vi "Convolutional_perso.vi"() -> ()   [LabVIEW 2018]
uses:
  <vilib>/Analysis/1siggen.llb/Ramp Pattern by Samples.vi
  <vilib>/addons/Modulation/Digital/General/MT Generate Bits (Galois, PN Order).vi
  <vilib>/addons/Modulation/Digital/Channel Coding/MT Convolutional Encoder (Rate).vi
  <vilib>/Analysis/baseanly.llb/Mean (DBL).vi
  <vilib>/addons/Modulation/Analog/support/mod_Set Error Source.vi
  <vilib>/addons/Modulation/Digital/Support/Common/Validators/mod_Generate Bits Validate.vi
  <vilib>/addons/Modulation/Digital/Support/Common/Validators/mod_Validate Bit Stream.vi
  <vilib>/addons/Modulation/Digital/Channel Coding/Convolutional codes/mod_Convolutional encoder.vi
  <vilib>/addons/Modulation/Digital/Support/Common/Validators/mod_AWGN Validate.vi
  <vilib>/addons/Modulation/Digital/Impairments/subVIs/mod_createSeeds.vi
  <vilib>/addons/Modulation/Digital/Channel Coding/Convolutional codes/subVIs/mod_Generate encoder tap connections.vi
  <vilib>/addons/Modulation/Digital/Channel Coding/Convolutional codes/subVIs/mod_Perform convolutional encoding.vi
  <vilib>/addons/Modulation/Digital/Channel Coding/Block codes/subVIs/mod_Buffer block code info (I8).vi
  <vilib>/addons/Modulation/Digital/Channel Coding/Convolutional codes/subVIs/mod_Generate valid reset (convolutional, I8).vi
  <vilib>/addons/Modulation/Digital/Support/Common/Validators/mod_Validate Samples Per Symbol.vi
  <vilib>/addons/Modulation/Analog/support/Validators/mod_Validate Complex Waveform.vi
  <vilib>/addons/Modulation/Analog/support/Validators/mod_WFErrorHandler.vi
  <vilib>/addons/Modulation/Digital/Support/Common/Validators/mod_Generate Filter Coefficients Validate.vi
  <vilib>/addons/Modulation/Digital/General/subVIs/mod_Generate Filter Coefficients.vi
  <vilib>/addons/Modulation/Digital/General/MT Generate PSK System Parameters(M).vi
  <vilib>/addons/Modulation/Digital/General/subVIs/mod_Generate Bits PN Sequence.vi
  <vilib>/addons/Modulation/Digital/Channel Coding/Convolutional codes/subVIs/mod_Select known generator matrix.vi
  <vilib>/addons/Modulation/Digital/Support/Common/Validators/mod_Validate Convolutional Encoder prms.vi
  <vilib>/Analysis/1siggen.llb/Gaussian White Noise (obs 90).vi
  <vilib>/addons/Modulation/Digital/General/MT Apply Matched Filter (Generic).vi
  <vilib>/addons/Modulation/Digital/General/MT Map PSK Symbols to Bits.vi
  <vilib>/addons/Modulation/Digital/Channel Coding/MT Convolutional Decoder (Viterbi Hard Decision, Rate).vi
  <vilib>/addons/Modulation/Digital/Demodulation/MT Calculate BER After Trigger (PN Sequence).vi
  <vilib>/addons/Modulation/niDMT.lvlib
  <vilib>/Analysis/NI_AALBase.lvlib
panel:
  out "size(s) 2":i32
  out "size(s)":i32
  out "Y":cdb[](array[numeric])
  out "error IO":errorcluster
  out "symbol map":cdb[](array[numeric])
  in  "Traceback Depth (D)":i32=20
  in  "Constraint Length (K)":i32=3
  in  "Rate (k/n)":enum16{"1/2", "1/3", "1/4", "2/3", "3/4"}(ring)
  in  "PN Sequence Order":i32=19
  in  "Seed In":i32=-1
  out "BER vs Eb/N0 (dB)\n[AWGN channel]":cluster{"Ramp Pattern":dbl[], dbl[]}(graph)
  in  "Trials per Eb/N0 Sample":i32=1
  in  "Start Eb/N0 (dB)":dbl=5.0 format="%0.2f"
  in  "End Eb/N0 (dB)":dbl=10.0 format="%0.2f"
  in  "Eb/N0 Samples":i32=6
  out "Progress in current trial":i32(slide) scale=0.0..100.0
  out "Accumulated BER (coding)":dbl format="%.4p"
  out "Current trial":i32
  out "Current Eb/N0":dbl
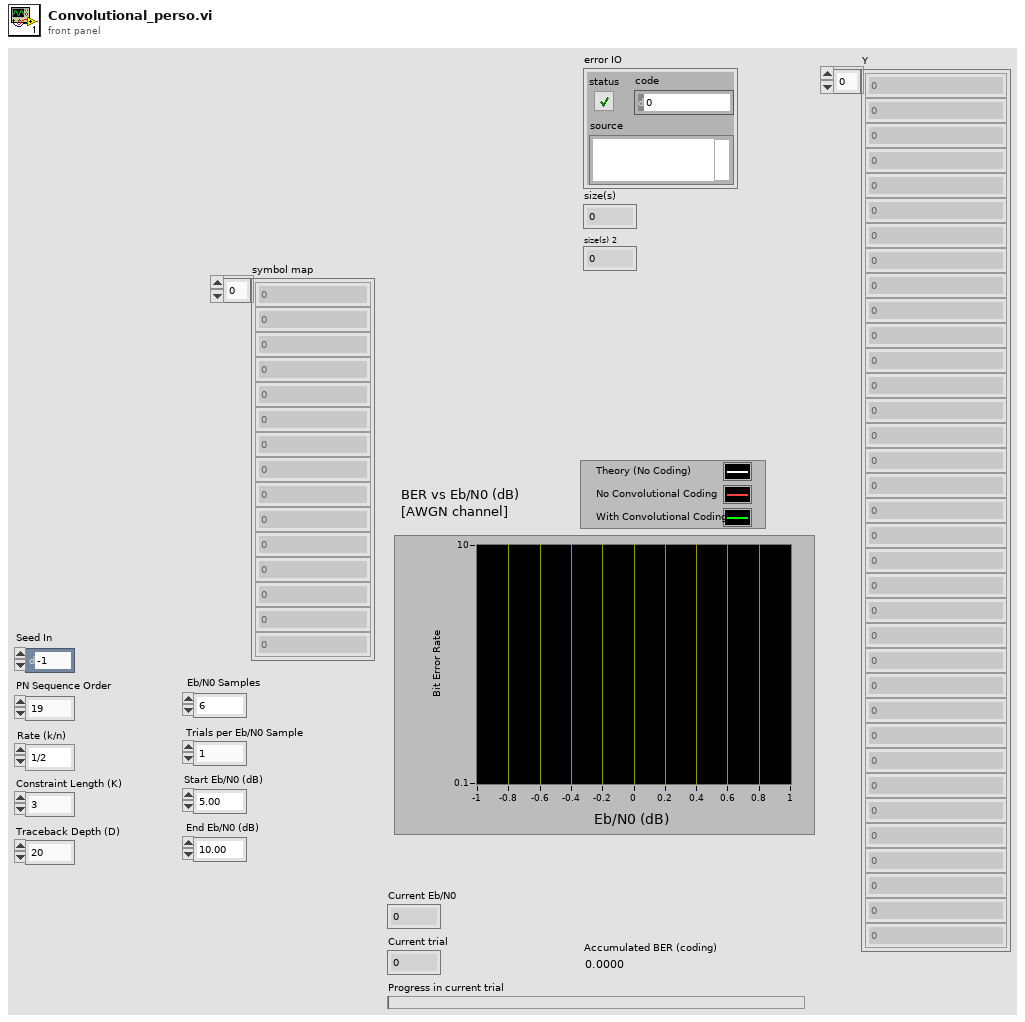
[diagram p1: front panel]
types:
  T1 = enum16{"none", "Raised Cosine", "Root Raised Cos", "Gaussian"}
  T2 = cluster{"samples per symbol (16)":i32, "symbol map":cdb[], "differential PSK":enum16{"disable", "enable"}, "PSK type":u16}
  T3 = typedef "niAMT.lvlib/Complex Data Waveform.ctl" = cluster{"t0":dbl, "dt":dbl, "Y":cdb[]}
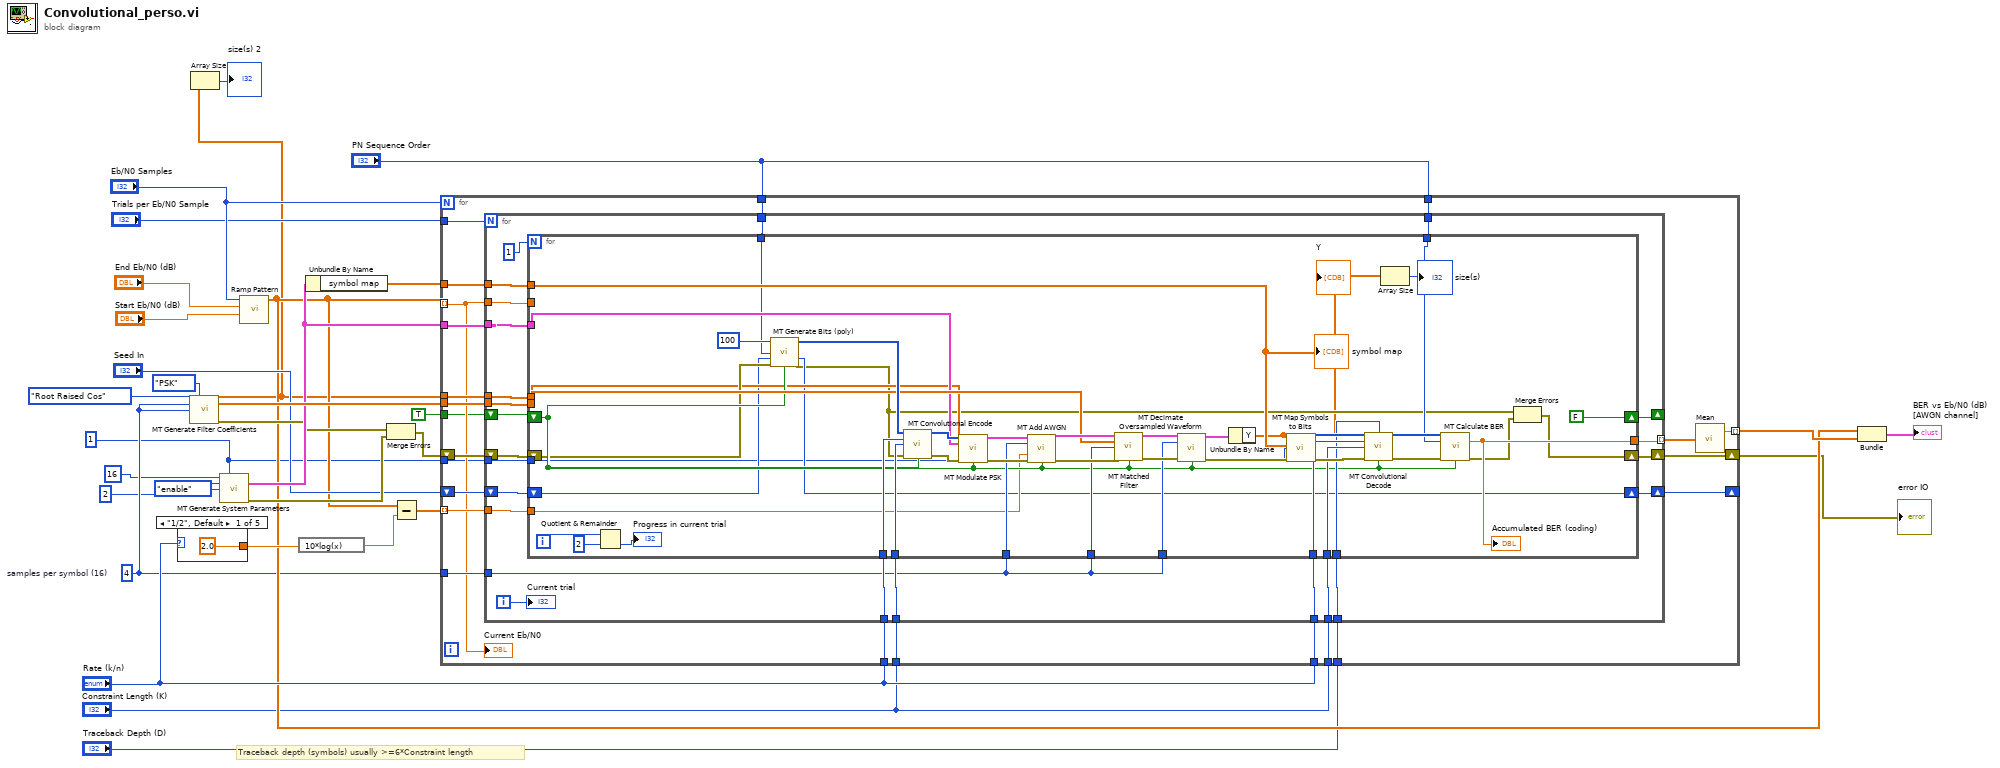
[diagram p0: block diagram]
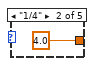
[diagram p2: hidden frame]
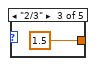
[diagram p3: hidden frame]
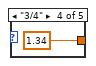
[diagram p4: hidden frame]
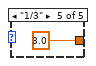
[diagram p5: hidden frame]
diagram:
  w3 = 1
  w8 = 4  # samples per symbol (16)
  # "Traceback depth (symbols) usually >=6*Constraint length"
  n1 = case shown="\"1/2\", Default" "Rate (k/n)" {
    tunnel: [2.0 4.0 1.5 1.34 3.0] -> w15
    frame "1/2", Default {
    }
    frame "1/4" {
    }
    frame "2/3" {
    }
    frame "3/4" {
    }
    frame "1/3" {
    }
  }
  n2 = call <vilib>:"MT Generate Filter Coefficients.vi"("pulse shaping filter (none)"=T1."Root Raised Cos", "modulation type"=enum16{"FSK", "PSK", "QAM", "MSK", "PAM", "ASK"}."PSK", "pulse shaping samples per symbol (16)"=w8, "matched samples per symbol (16)"=w8) -> ("pulse shaping filter coefficients"=w2:dbl[], "matched filter coefficients"=w28:dbl[], "error out"=w23:errorcluster)  [unwired: 9 in]
  n3 = Array Size(array=w2) -> (size(s)=→"size(s) 2":i32)
  n4 = call-poly <vilib>:"MT Generate System Parameters.vi"("samples per symbol (16)"=16, "PSK type"=w3, "M-PSK (4)"=2, "differential PSK"=enum16{"disable", "enable"}."enable") -> ("PSK system parameters"=w27:T2, "error out"=w22:errorcluster)  [unwired: 9 in, 1 out]
  n5 = call-poly <vilib>:"Ramp Pattern.vi"("start"="Start Eb/N0 (dB)", "end"="End Eb/N0 (dB)", "samples"="Eb/N0 Samples") -> ("Ramp Pattern"=w13:dbl[])  [unwired: 7 in, 1 out]
  n6 = expression code="10*log(x)"(w15) -> (w14:dbl)
  n7 = Unbundle By Name(w27) -> ("symbol map"=w26:cdb[])
  n8 = Merge Errors(w23, w22) -> (w21:errorcluster)
  n9 = Subtract(x=w13, y=w14) -> (x-y=w20:dbl[])
  n10 = for {
    N: "Eb/N0 Samples" -> [_]
    tunnel: w2 -> [w60]
    tunnel: "Rate (k/n)" -> [w58]
    tunnel: "Constraint Length (K)" -> [w57]
    tunnel: w13 -> [w40] mode=indexing
    tunnel: w28 -> [w56]
    tunnel: w8 -> [w55]
    tunnel: w26 -> [w54]
    tunnel: "Rate (k/n)" -> [w53]
    tunnel: "Constraint Length (K)" -> [w52]
    tunnel: "Traceback Depth (D)" -> [w51]
    tunnel: "Trials per Eb/N0 Sample" -> [w50]
    tunnel: [w48] -> w17 mode=indexing
    tunnel: w27 -> [w59]
    shift-right: [w47] -> w4
    shift-left: w21 -> [w46]
    tunnel: w20 -> [w45] mode=indexing
    shift-right: [w43] -> _
    shift-left: "Seed In" -> [w44]
    tunnel: "PN Sequence Order" -> [w42]
    tunnel: "PN Sequence Order" -> [w41]
    tunnel: TRUE ("reset? (T)") -> [w39]
    tunnel: w3 -> [w38]
    n11 = for {
      N: w50 -> [_]
      tunnel: w60 -> [w84]
      tunnel: w58 -> [w82]
      tunnel: w57 -> [w81]
      tunnel: w40 -> [w80]
      tunnel: w56 -> [w79]
      tunnel: w55 -> [w78]
      tunnel: w54 -> [w77]
      tunnel: w53 -> [w76]
      tunnel: w52 -> [w75]
      tunnel: w51 -> [w74]
      tunnel: [w72] -> w49 mode=indexing
      tunnel: w59 -> [w83]
      shift-right: [w70] -> w47
      shift-left: w46 -> [w69]
      tunnel: w45 -> [w68]
      shift-right: [w66] -> w43
      shift-left: w44 -> [w67]
      tunnel: w42 -> [w65]
      tunnel: w41 -> [w64]
      shift-right: [w62] -> _
      shift-left: w39 -> [w63]
      tunnel: w38 -> [w61]
      i -> [w71]
      n12 = for {
        N: 1 -> [_]
        tunnel: w84 -> [w97]
        shift-right: [FALSE ("reset? (T)")] -> w62
        shift-left: w63 -> [w103]
        tunnel: w82 -> [w126]
        tunnel: w81 -> [w125]
        tunnel: w80 -> [_]
        tunnel: w79 -> [w122]
        tunnel: w78 -> [w116]
        tunnel: w78 -> [w114]
        tunnel: w78 -> [w115]
        tunnel: w77 -> [w112]
        tunnel: w76 -> [w108]
        tunnel: w75 -> [w107]
        tunnel: w74 -> [w106]
        tunnel: [w101] -> w72
        tunnel: w83 -> [w119]
        shift-right: [w99] -> w70
        shift-left: w69 -> [w98]
        tunnel: w68 -> [w96]
        shift-right: [w94] -> w66
        shift-left: w67 -> [w95]
        tunnel: w65 -> [w93]
        tunnel: w64 -> [w92]
        tunnel: w61 -> [w87]
        i -> [w90]
        n13 = Quotient & Remainder(x=w90, y=2) -> (floor(x/y)=→"Progress in current trial":i32)  [unwired: 1 out]
        n14 = call-poly <vilib>:"MT Generate Bits (poly).vi"("total bits (128)"=100, "PN sequence order (9)"=w93, "seed in (0xD6BF7DF2)"=w95, "error in (no error)"=w98, "reset? (T)"=w103) -> ("output bit stream"=w127:i8[], "seed out"=w94:i32, "error out"=w88:errorcluster)  [unwired: 8 in]
        n15 = call-poly <vilib>:"MT Convolutional Encode.vi"("input bit stream"=w127, "rate (k/n)"=w126, "constraint length (K)"=w125, "error in (no error)"=w88, "reset? (T)"=w103) -> ("output bit stream"=w128:i8[], "error out"=w120:errorcluster)  [unwired: 8 in, 1 out]
        n16 = call <vilib>:"MT Modulate PSK.vi"("input bit stream"=w128, "PSK system parameters"=w119, "pulse shaping filter coefficients"=w97, "error in (no error)"=w120, "reset? (T)"=w103) -> ("output complex waveform"=w129:T3, "error out"=w121:errorcluster)  [unwired: 8 in, 1 out]
        n17 = call <vilib>:"MT Add AWGN.vi"("input complex waveform"=w129, "samples per symbol (16)"=w115, "Eb/N0 (10 dB)"=w96, "error in (no error)"=w121, "reset? (T)"=w103) -> ("output complex waveform"=w123:T3, "error out"=w124:errorcluster)  [unwired: 8 in, 1 out]
        n18 = call-poly <vilib>:"MT Matched Filter.vi"("input complex waveform"=w123, "matched filter coefficients"=w122, "samples per symbol (16)"=w114, "error in (no error)"=w124, "reset? (T)"=w103) -> ("output complex waveform"=w118:T3, "error out"=w117:errorcluster)  [unwired: 9 in]
        n19 = call <vilib>:"MT Decimate Oversampled Waveform.vi"("input complex waveform"=w118, "decimation factor"=w116, "error in (no error)"=w117, "reset? (T)"=w103) -> ("output complex waveform"=w111:T3, "error out"=w113:errorcluster)  [unwired: 10 in]
        n20 = Unbundle By Name(w111) -> ("Y"=w86:cdb[])
        "Y" <- w86
        n21 = call-poly <vilib>:"MT Map Symbols to Bits.vi"("symbols"=w86, "symbol map"=w112, "PSK type"=w87, "error in (no error)"=w113) -> ("output bit stream"=w109:i8[], "error out"=w110:errorcluster)  [unwired: 10 in]
        n22 = call-poly <vilib>:"MT Convolutional Decode.vi"("input bit stream"=w109, "traceback depth (D)"=w106, "rate (k/n)"=w108, "constraint length (K)"=w107, "error in (no error)"=w110, "reset? (T)"=w103) -> ("output bit stream"=w104:i8[], "error out"=w105:errorcluster)  [unwired: 7 in, 1 out]
        n23 = Array Size(array=w86) -> (size(s)=→"size(s)":i32)
        n24 = call-poly <vilib>:"MT Calculate BER.vi"("input bit stream"=w104, "PN sequence order (9)"=w92, "error in (no error)"=w105, "reset? (T)"=w103) -> ("accumulated BER"=w101:dbl, "error out"=w100:errorcluster)  [unwired: 7 in, 3 out]
        "Accumulated BER (coding)" <- w101
        n25 = Merge Errors(w88, w100) -> (w99:errorcluster)
        "symbol map" <- w112
      }
      "Current trial" <- w71
    }
    n26 = call-poly <vilib>:"Mean.vi"("X"=w49) -> ("mean"=w48:dbl)  [unwired: 1 out]
    "Current Eb/N0" <- w40
  }
  "error IO" <- w4
  n27 = Bundle("Ramp Pattern"=w13, w17) -> (→"BER vs Eb/N0 (dB)\n[AWGN channel]":cluster{"Ramp Pattern":dbl[], dbl[]})  [unwired: 1 in]
